vi "WildBugChilGru_V0.195.vi"() -> ()   [LabVIEW 2014]
uses:
  <vilib>/Utility/miscctls.llb/LVPointTypeDef.ctl
  <vilib>/Analysis/NI_AALBase.lvlib
  <vilib>/gmath/NI_Gmath.lvlib
  <vilib>/Analysis/NI_AALPro.lvlib
  <vilib>/Utility/xml.llb/Read From XML File(string).vi
  <vilib>/Utility/xml.llb/Write to XML File(string).vi
  <vilib>/Instr/_visa.llb/VISA Configure Serial Port (Instr).vi
  <vilib>/Analysis/3filter.llb/IIR Filter (DBL).vi
panel:
  in  "Registerkarte":T1(tab)
  in  "Gleitender Mittelwert":u8=35
  in  "Differenzenquotient":u8=12
  in  "Polynom":u8=15
  in  "n vom Gas [1/min]":dbl=5000.0
  in  "Zündung [Imp/U]":u8=5
  in  "Übersetzung ermitteln aus":T2(ring)
  in  "Getriebe [1:]":dbl=5.343
  in  "Reifenumfang [m]":dbl=1.222
  in  "Dauer [s]":dbl=5.0
  in  "nKuWe/nRolle":dbl=10.0
  in  "Rolle [Inkr/U]":u16=10
  in  "Rollenumfang [m]":dbl=0.613
  in  "Rollenträgheit [kgm²]":dbl=0.402
  in  "Lufttemperatur [°C]":dbl=20.0
  in  "Luftfeuchtigkeit [%]":dbl=50.0
  in  "Luftdruck [mbar]":dbl=1013.0
  in  "Messung Klimadaten":bool
  in  "Recalc":bool
  in  "Ende":bool
  out "Datenspeicher":T3
  out "COM-Fehlerrate":string="0 / 0,0%"
  in  "Konfiguration:":bool
  in  "Speichern":bool
  in  "Drucken":bool
  out "Pmax":string="0,0 PS"
  out "Ergebnis":string="0,0 PS bei 0 1/min   |   0,0 Nm bei 0 1/min   |   vmax: 2147483647 km/h\nDIN 70020 k =1,000 (20 °C, 50 %, 1013 mbar)\n20.11.2016 20:05 "
  in  "Fahrzeugdaten":string="Hier die Fahrzeugdaten eingeben"
  out "XY-Graph":cluster{dbl[], dbl[]}[](graph)
  out "Untersetzung\nermittelt":bool
  out "Untersetzung":dbl format="%#.2f"
  in  "Start [F1]":bool
  out "Füllstand Lesepuffer":u64(slide) scale=1.0..100.0
  out "Hinterrad\n[km/h]":dbl(knob) scale=0.0..150.0
  out "Welle\n[1/min]":cluster{dbl, dbl}(knob) scale=0.0..12000.0
  out "Lesepuffer":string="\n"
  in  "Serielle Schnittstelle":refnum<visa-resource-name>="COM6"
  out "Untersetzung-Graph":dbl(graph)=2.6802446808510636 caption="Untersetzung"
  # "1. n konstant halten\n2. START\n3. n weiter halten\n4. bei GO: Vollgas\n5. vom Gas gehen"
  # "Zündung\nRolle"
  # "Untersetzung aus:"
  # "Eingabe <> Messen"
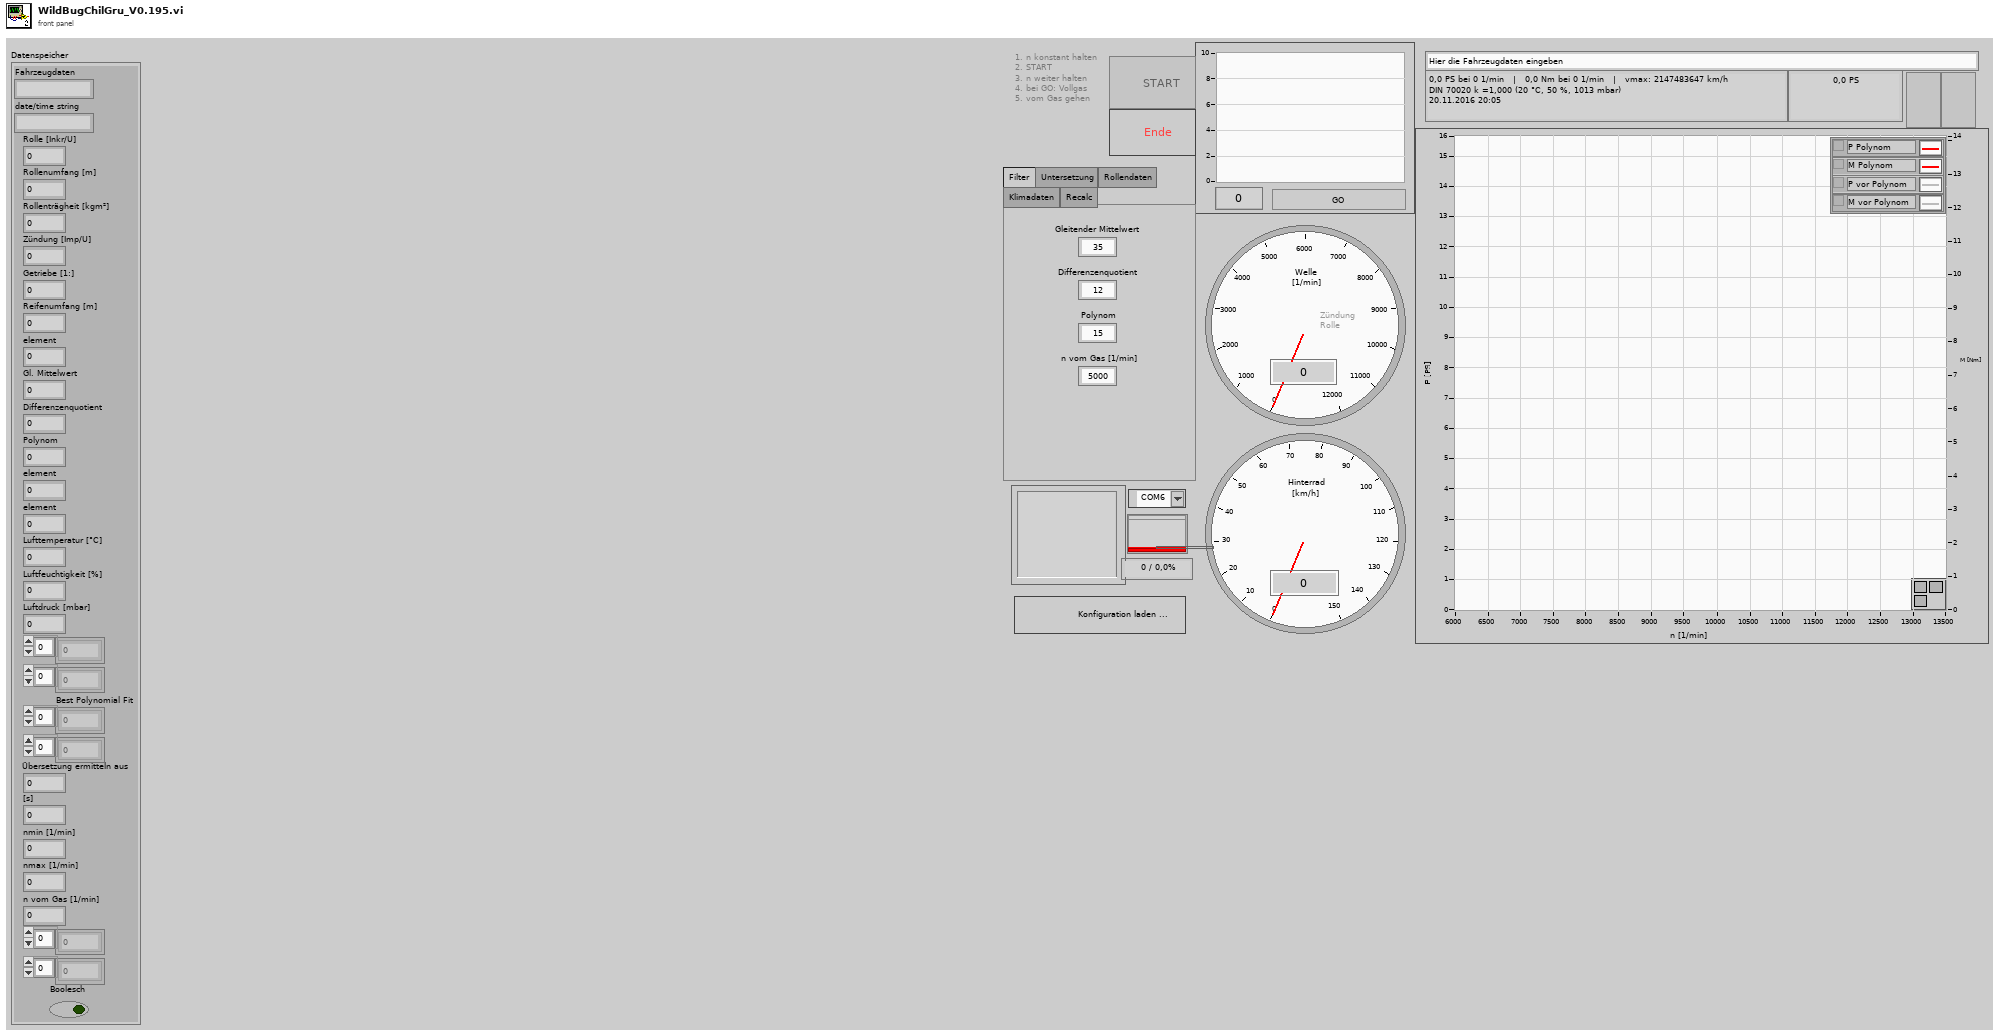
[diagram p1: front panel]
types:
  T1 = enum32{"Filter", "Untersetzung", "Rollendaten", "Klimadaten", "Recalc"}
  T2 = enum8{"Zündsignal", "Getriebe & Reifen", "nKuWe / nRolle"}
  T3 = cluster{"Fahrzeugdaten":string, "date/time string":string, "Rolle [Inkr/U]":u16, "Rollenumfang [m]":dbl, "Rollenträgheit [kgm²]":dbl, "Zündung [Imp/U]":u8, "Getriebe [1:]":dbl, "Reifenumfang [m] ":dbl, "element":dbl, "Gl. Mittelwert":u8, "Differenzenquotient":u8, "Polynom":u8, "element":dbl, "element":dbl, "Lufttemperatur [°C]":dbl, "Luftfeuchtigkeit [%]":dbl, "Luftdruck [mbar]":dbl, dbl[], dbl[], "Best Polynomial Fit":dbl[], dbl[], "Übersetzung ermitteln aus":u8, "[s]":dbl, "nmin [1/min]":dbl, "nmax [1/min]":dbl, "n vom Gas [1/min]":dbl, dbl[], i32[], "Boolesch":bool}
  T4 = enum16{"Kleinste Quadrate", "Kleinestes absolutes Reiduum", "Biquadrat"}
  T5 = enum8{"Enabled", "Disabled", "Disabled and Grayed Out"}
  T6 = cluster{"Fahrzeugdaten":string, "date/time string":string, "Rolle [Inkr/U]":u16, "Rollenumfang [m]":dbl, "Rollenträgheit [kgm²]":dbl, "Zündung [Imp/U]":u8, "Getriebe [1:]":dbl, "Reifenumfang [m] ":dbl, "mean value":dbl, "Gleitender Mittelwert":u8, "Differenzenquotient":u8, "Polynom":u8, dbl, "element":dbl, "Lufttemperatur [°C]":dbl, "Luftfeuchtigkeit [%]":dbl, "Luftdruck [mbar]":dbl, dbl[], dbl[], "Best Polynomial Fit":dbl[], dbl[], "Übersetzung ermitteln aus":enum8{"Zündsignal", "Getriebe & Reifen", "nKuWe / nRolle"}, "Dauer [s]":dbl, dbl, dbl, "n vom Gas [1/min]":dbl, dbl[], i32[], "Messung Klimadaten":bool}
  T7 = typedef "LVPointTypeDef.ctl" = cluster{"Horizontal":i16, "Vertical":i16}
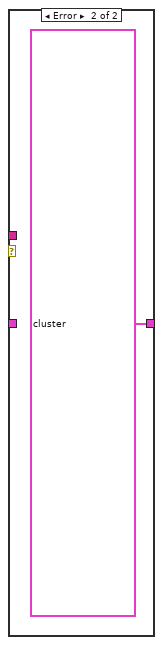
[diagram p2: hidden frame]
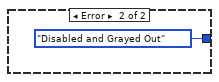
[diagram p3: hidden frame]
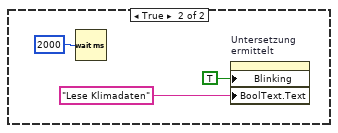
[diagram p5: hidden frame]
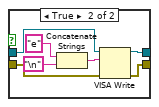
[diagram p6: hidden frame]
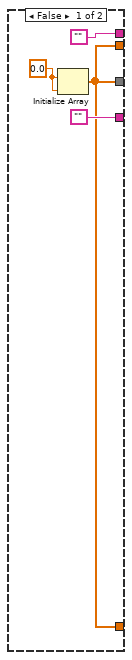
[diagram p8: hidden frame]
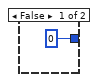
[diagram p9: hidden frame]
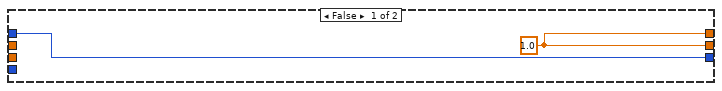
[diagram p11: hidden frame]
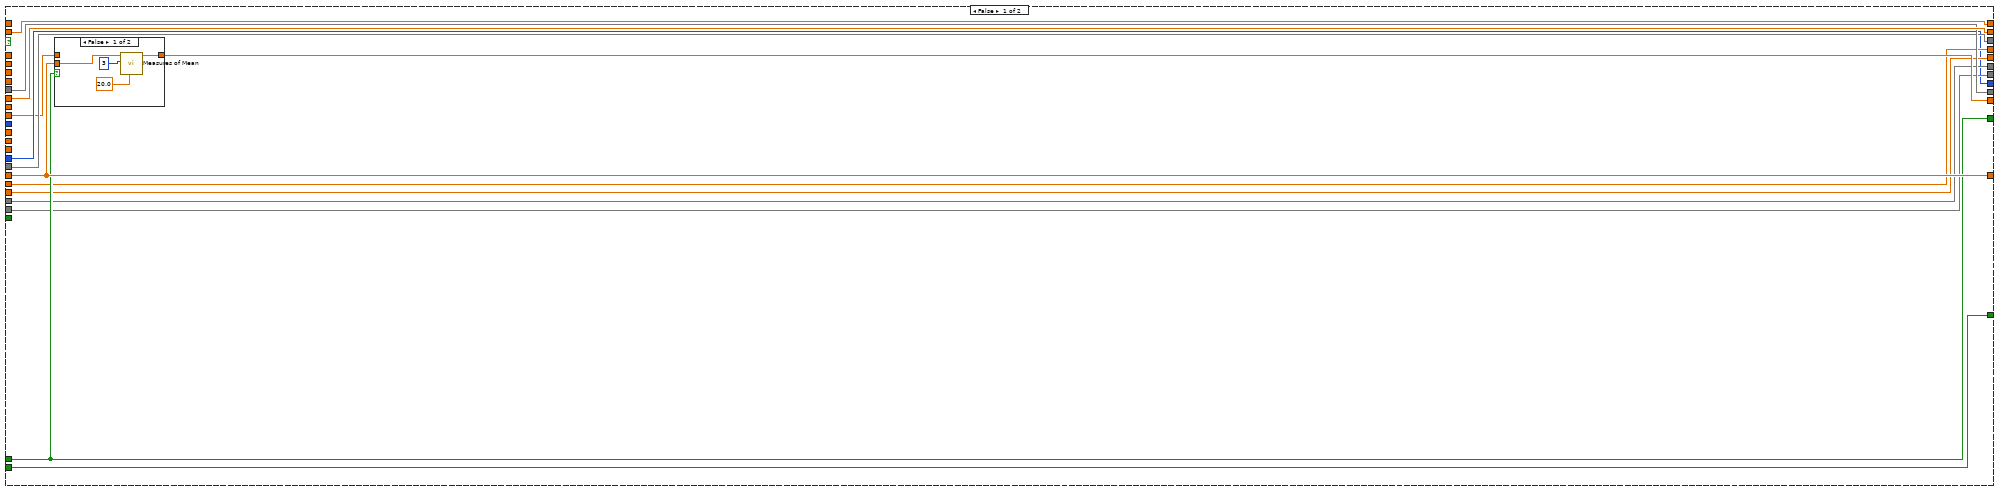
[diagram p12: hidden frame]
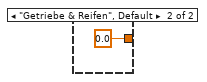
[diagram p16: hidden frame]
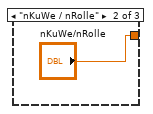
[diagram p18: hidden frame]
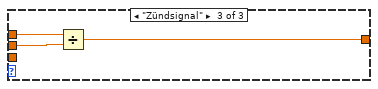
[diagram p19: hidden frame]
diagram:
  n1 = while {
    stop <- w1 stop-if-true
    n2 = event shown="[0] \"Start [F1]\": Wertänderung" {
      selector: _ -> [_ _]
      dyn-events: _ -> [_ _]
      timeout: _ -> [_ _]
      tunnel: [_ TRUE] -> w1
      event "Start [F1]": Value Change {
        n3 = event-data() -> ("NewVal"=w2:bool)  [unwired: 1 in, 5 out]
        n4 = case shown="True" w2 {
          frame False {
          }
          frame True {
            n5 = flat-sequence {
              tunnel: [w132] -> w117
              tunnel: [w131] -> w116
              tunnel: ["Messung Klimadaten"] -> w115
              tunnel: w117 -> [w145]
              tunnel: w116 -> [w144]
              tunnel: [0] -> w114
              tunnel: [1.0 ("element")] -> w113
              tunnel: [w142] -> w112
              tunnel: [w156] -> w111
              tunnel: [0] -> w110
              tunnel: [w142] -> w109
              tunnel: [-5] -> w108
              tunnel: [w153] -> w107
              tunnel: [w151] -> w106
              tunnel: [w150] -> w105
              tunnel: [0.0] -> w104
              tunnel: [w145] -> w103
              tunnel: [w144] -> w102
              tunnel: w115 -> [w143]
              tunnel: [w143] -> w101
              tunnel: w114 -> [w182]
              tunnel: [w182] -> w100
              tunnel: w113 -> [w181]
              tunnel: [w181] -> w99
              tunnel: w112 -> [w180]
              tunnel: [w180] -> w98
              tunnel: w111 -> [w179]
              tunnel: [w179] -> w97
              tunnel: w110 -> [w178]
              tunnel: [w178] -> w96
              tunnel: w109 -> [w177]
              tunnel: [w177] -> w95
              tunnel: w108 -> [w176]
              tunnel: [w176] -> w94
              tunnel: w107 -> [w175]
              tunnel: [w175] -> w93
              tunnel: w106 -> [w174]
              tunnel: [w174] -> w92
              tunnel: w105 -> [w173]
              tunnel: [w173] -> w91
              tunnel: w104 -> [w172]
              tunnel: [w172] -> w90
              tunnel: w103 -> [w171]
              tunnel: [w168] -> w89
              tunnel: w102 -> [w170]
              tunnel: [w169] -> w88
              tunnel: [w167] -> w87
              tunnel: w101 -> [w167]
              tunnel: w100 -> [w206]
              tunnel: [w206] -> w86
              tunnel: w99 -> [w205]
              tunnel: [w205] -> w85
              tunnel: w98 -> [w204]
              tunnel: [w204] -> w84
              tunnel: w97 -> [w203]
              tunnel: [w203] -> w83
              tunnel: w96 -> [w202]
              tunnel: [w202] -> w82
              tunnel: w95 -> [w201]
              tunnel: [w201] -> w81
              tunnel: w94 -> [w200]
              tunnel: [w200] -> w80
              tunnel: w93 -> [w199]
              tunnel: [w199] -> w79
              tunnel: w92 -> [w198]
              tunnel: [w198] -> w78
              tunnel: w91 -> [w197]
              tunnel: [w197] -> w77
              tunnel: w90 -> [w196]
              tunnel: [w196] -> w76
              tunnel: w89 -> [w195]
              tunnel: [w195] -> w75
              tunnel: w88 -> [w194]
              tunnel: [w194] -> w74
              tunnel: w87 -> [w192]
              tunnel: [w192] -> w73
              tunnel: w86 -> [w222]
              tunnel: [w222] -> w72
              tunnel: w85 -> [w221]
              tunnel: [w221] -> w71
              tunnel: w84 -> [w220]
              tunnel: [w220] -> w70
              tunnel: w83 -> [w219]
              tunnel: [w219] -> w69
              tunnel: w82 -> [w218]
              tunnel: [w218] -> w68
              tunnel: w81 -> [w217]
              tunnel: [w217] -> w67
              tunnel: w80 -> [w216]
              tunnel: [w216] -> w66
              tunnel: w79 -> [w215]
              tunnel: [w215] -> w65
              tunnel: w78 -> [w214]
              tunnel: [w214] -> w64
              tunnel: w77 -> [w213]
              tunnel: [w213] -> w63
              tunnel: w76 -> [w212]
              tunnel: [w212] -> w62
              tunnel: w75 -> [w211]
              tunnel: [w210] -> w61
              tunnel: w74 -> [w208]
              tunnel: [w209] -> w60
              tunnel: w73 -> [w207]
              tunnel: w72 -> [w296]
              tunnel: w71 -> [w295]
              tunnel: w70 -> [w294]
              tunnel: w69 -> [w293]
              tunnel: w68 -> [w292]
              tunnel: w67 -> [w291]
              tunnel: w66 -> [w290]
              tunnel: w65 -> [w289]
              tunnel: w64 -> [w288]
              tunnel: w63 -> [w287]
              tunnel: w62 -> [w286]
              tunnel: w61 -> [w251]
              tunnel: [w296] -> w59
              tunnel: [w295] -> w58
              tunnel: [w294] -> w57
              tunnel: [w293] -> w56
              tunnel: [w292] -> w55
              tunnel: [w291] -> w54
              tunnel: [w290] -> w53
              tunnel: [w289] -> w52
              tunnel: [w288] -> w51
              tunnel: [w287] -> w50
              tunnel: [w286] -> w49
              tunnel: [w251] -> w48
              tunnel: [w250] -> w47
              tunnel: [w285] -> w46
              tunnel: [w284] -> w45
              tunnel: [w283] -> w44
              tunnel: ["Gleitender Mittelwert"] -> w43
              tunnel: w60 -> [w250]
              tunnel: [w305] -> w9
              tunnel: [w306] -> w10
              tunnel: [w307] -> w11
              tunnel: [w308] -> w12
              tunnel: [w299] -> w7
              tunnel: [w298] -> w8
              tunnel: [w309] -> w13
              tunnel: [w310] -> w14
              tunnel: [w311] -> w16
              tunnel: [w312] -> w18
              tunnel: [w313] -> w19
              tunnel: [w314] -> w20
              tunnel: [w315] -> w37
              tunnel: [w316] -> w39
              tunnel: [w317] -> w40
              tunnel: [w318] -> w41
              tunnel: [w319] -> w42
              tunnel: w59 -> [w319]
              tunnel: w58 -> [w318]
              tunnel: w57 -> [w317]
              tunnel: w56 -> [w316]
              tunnel: w55 -> [w315]
              tunnel: w54 -> [w314]
              tunnel: w53 -> [w313]
              tunnel: w52 -> [w312]
              tunnel: w51 -> [w311]
              tunnel: w50 -> [w310]
              tunnel: w49 -> [w309]
              tunnel: w48 -> [w301]
              tunnel: w47 -> [w300]
              tunnel: w46 -> [w308]
              tunnel: w45 -> [w307]
              tunnel: w44 -> [w306]
              tunnel: w43 -> [w305]
              frame #0 {
                w137 = u16 0 items=["None", "XON/XOFF", "RTS/CTS", "XON/XOFF & RTS/CTS", "DTR/DSR", "XON/XOFF & DTR/DSR"] ("flow control (0:none)")
                w138 = u16 10 items=["1.0"=10, "1.5"=15, "2.0"=20] ("stop bits (10: 1 bit)")
                w130 = FALSE  # Enable Termination Char (T)
                w133 = u32 10000  # timeout (10sec)
                n6 = call-poly "VISA Configure Serial Port"("VISA resource name"="Serielle Schnittstelle", "timeout (10sec)"=w133, "Enable Termination\nChar (T)"=w130, "baud rate (9600)"=u32 250000 ("baudrate (250000)"), "data bits (8)"=u16 8, "parity (0:none)"=enum16{"None", "Odd", "Even", "Mark", "Space"}."None", "stop bits (10: 1 bit)"=w138, "flow control (0:none)"=w137) -> ("VISA resource name out"=w135:refnum<visa-resource-name>, "error out"=w134:errorcluster)  [unwired: 6 in]
                n7 = VISA Clear(VISA resource name=w135, error in (no error)=w134) -> (VISA resource name out=w132:refnum<visa-resource-name>, error out=w131:errorcluster)
              }
              frame #1 {
                w146 = T5."Disabled and Grayed Out" ("Deaktiviert")
                w149 = 0.0  # Graphen löschen
                w152 = 0
                w157 = 0.0
                w142 = FALSE
                w150 = ""
                n8 = case shown="False" w143 {
                  frame False {
                    n9 = property on="Untersetzung\nermittelt" class="Bool. (strikt)"("Blinking"=TRUE ("Blinkend"), "BoolText.Text"="Initialisiere" ("Beschriftung.Text")) -> ()  [unwired: 2 in, 2 out]
                  }
                  frame True {
                    n10 = Wait (ms)(milliseconds to wait=u32 2000 ("Zu wartende ms")) -> ()  [unwired: 1 out]
                    n11 = property on="Untersetzung\nermittelt" class="Bool. (strikt)"("Blinking"=TRUE ("Blinkend"), "BoolText.Text"="Lese Klimadaten" ("Beschriftung.Text")) -> ()  [unwired: 2 in, 2 out]
                  }
                }
                n12 = Build Array(w149) -> (w148:dbl[])
                n13 = property on="Drucken" class="Bool. (strikt)"("DisabledEnum"=w146) -> ()  [unwired: 2 in, 2 out]
                n14 = property on="Übersetzung ermitteln aus" class="Enum (strikt)"("DisabledEnum"=w146) -> ()  [unwired: 2 in, 2 out]
                n15 = property on="Konfiguration:" class="Bool. (strikt)"("DisabledEnum"=w146) -> ()  [unwired: 2 in, 2 out]
                n16 = property on="Ende" class="Bool. (strikt)"("DisabledEnum"=w146) -> ()  [unwired: 2 in, 2 out]
                n17 = property on="Speichern" class="Bool. (strikt)"("DisabledEnum"=w146) -> ()  [unwired: 2 in, 2 out]
                n18 = property on="Untersetzung-Graph" class="SVDiagr (strikt)"("History Data"=w148) -> ()  [unwired: 2 in, 2 out]
                n19 = local write "Pmax"(w150) -> ()
                n20 = local write "COM-Fehlerrate"(w150) -> ()
                n21 = local write "Ergebnis"(w150) -> ()
                n22 = Initialize Array(w157, w157) -> (w156:dbl[])
                n23 = Initialize Array(w152, w152) -> (w151:i32[])
                n24 = Initialize Array(0.0 ("y"), 0) -> (w153:dbl[])
              }
              frame #2 {
                n25 = case shown="False" w167 {
                  tunnel: w171 -> [w184 w188]
                  tunnel: w170 -> [w183 w187]
                  tunnel: [w183 w186] -> w169
                  tunnel: [w184 w185] -> w168
                  frame False {
                  }
                  frame True {
                    n26 = Concatenate Strings("e" ("String"), "\n") -> (w191:string)
                    n27 = VISA Write(VISA resource name=w188, write buffer=w191, error in (no error)=w187) -> (VISA resource name out=w185:refnum<visa-resource-name>, error out=w186:errorcluster)  [unwired: 1 out]
                  }
                }
              }
              frame #3 {
                n28 = Wait (ms)(milliseconds to wait=u32 500 ("Zu wartende ms")) -> ()  [unwired: 1 out]
              }
              frame #4 {
                n29 = case shown="True" w207 {
                  tunnel: w211 -> [w224 w245]
                  tunnel: [w224 w244] -> w210
                  tunnel: [w223 w243] -> w209
                  tunnel: w208 -> [w223 w242]
                  frame False {
                  }
                  frame True {
                    w227 = ";" ("Regulärer Ausdruck")
                    n30 = property class="Instr"(reference=w245, error in=w242) -> (reference out=w248:refnum<visa-resource-name>, error out=w247:errorcluster, "Serial Settings:Number of Bytes at Serial Port"=w246:u32)
                    n31 = VISA Read(VISA resource name=w248, byte count=w246, error in (no error)=w247) -> (VISA resource name out=w244:refnum<visa-resource-name>, read buffer=w239:string, error out=w243:errorcluster)  [unwired: 1 out]
                    n32 = Search and Replace String(replace all?=TRUE ("Alle ersetzen? (F)"), input string=w239, search string="." ("Such-String"), replace string="," ("Ersetzungs-String (\"\")")) -> (result string=w232:string)  [unwired: 4 in, 3 out]
                    n33 = Match Pattern(string=w232, regular expression=w227) -> (before substring=w230:string, after substring=w231:string)  [unwired: 1 in, 2 out]
                    n34 = Match Pattern(string=w231, regular expression=w227) -> (before substring=w229:string, after substring=w228:string)  [unwired: 1 in, 2 out]
                    n35 = Fract/Exp String To Number(string=w230, offset=1 ("Offset")) -> (number=w238:dbl)  [unwired: 2 in, 1 out]
                    n36 = local write "Lufttemperatur [°C]"(w238) -> ()
                    n37 = Fract/Exp String To Number(string=w229) -> (number=w235:dbl)  [unwired: 3 in, 1 out]
                    n38 = Match Pattern(string=w228, regular expression=w227) -> (before substring=w226:string)  [unwired: 1 in, 3 out]
                    n39 = Fract/Exp String To Number(string=w226) -> (number=w237:dbl)  [unwired: 3 in, 1 out]
                    n40 = Divide(x=w235, y=100.0 ("x")) -> (x/y=w236:dbl)
                    n41 = local write "Luftdruck [mbar]"(w236) -> ()
                    n42 = local write "Luftfeuchtigkeit [%]"(w237) -> ()
                  }
                }
              }
              frame #5 {
                n43 = Wait (ms)(milliseconds to wait=u32 2000 ("Zu wartende ms")) -> ()  [unwired: 1 out]
                n44 = Add(x="Lufttemperatur [°C]", y=273.15) -> (x+y=w266:dbl)
                n45 = Divide ("M_Welle [Nm]")(x=300.0, y=w266) -> (x/y=w269:dbl)
                n46 = Multiply(x="Luftfeuchtigkeit [%]", y=0.01) -> (x*y=w280:dbl)
                n47 = Divide ("M_Welle [Nm]")(x=w266, y=293.15) -> (x/y=w264:dbl)
                n48 = Multiply(x=w280, y=240800000000.0) -> (x*y=w254:dbl)
                n49 = Power Of X(1:w269, 2:5.0) -> (0:w267:dbl)
                n50 = Multiply(x=w254, y=w267) -> (x*y=w274:dbl)
                n51 = Multiply(x=w269, y=-22.644) -> (x*y=w275:dbl)
                n52 = Power Of X(1:w264, 2:0.5) -> (0:w261:dbl)
                n53 = Exponential(1:w275) -> (0:w273:dbl)
                n54 = Multiply(x=w274, y=w273) -> (x*y=w272:dbl)
                n55 = Subtract "p_Trocken [mbar]"(x="Luftdruck [mbar]", y=w272) -> (x-y=w270:dbl)
                n56 = Divide ("M_Welle [Nm]")(x=1013.0, y=w270) -> (x/y=w262:dbl)
                n57 = Multiply "Korrekturfaktor DIN 70020"(x=w262, y=w261) -> (x*y=w285:dbl)
                n58 = Divide(x="Gleitender Mittelwert", y=2) -> (x/y=w258:dbl)
                n59 = Round Toward -Infinity(1:w258) -> (0:w257:dbl)
                n60 = call <vilib>:"Smoothing Filter Coefficients.vi"("shape"=1, "half-width"=w257, "type"=0) -> ("forward coefficients"=w283:dbl[], "reverse coefficients"=w284:dbl[])  [unwired: 6 in, 1 out]
              }
              frame #6 {
                n61 = Concatenate Strings("m" ("String"), "\n") -> (w304:string)
                n62 = property on="Untersetzung\nermittelt" class="Bool. (strikt)"("Blinking"=FALSE ("Blinkend")) -> ()  [unwired: 2 in, 2 out]
                n63 = VISA Write(VISA resource name=w301, write buffer=w304, error in (no error)=w300) -> (VISA resource name out=w298:refnum<visa-resource-name>, error out=w299:errorcluster)  [unwired: 1 out]
              }
            }
            n64 = while {
              tunnel: w8 -> [w450]
              tunnel: w7 -> [w449]
              shift-right: [w520] -> _
              shift-left: w14 -> [w465]
              shift-right: [w515] -> _
              shift-left: w13 -> [w519]
              shift-right: [w514] -> _
              shift-left: w13 -> [w518]
              shift-right: [w469] -> _
              shift-left: w13 -> [w517]
              shift-right: [w496] -> _
              shift-left: w42 -> [w516]
              shift-right: [w457] -> w25
              shift-left: w41 -> [_]
              shift-right: [w475] -> w29
              shift-left: w13 -> [w497]
              shift-right: [w507] -> w27
              shift-left: w13 -> [w471]
              shift-right: [w470] -> _
              shift-left: w18 -> [w511]
              shift-right: [w508] -> _
              shift-left: w40 -> [w485]
              shift-right: [w451] -> _
              shift-left: w39 -> [_]
              shift-right: [w456] -> _
              shift-left: w39 -> [_]
              shift-right: [w506] -> w28
              shift-left: w39 -> [w504]
              shift-right: [w505] -> _
              shift-left: w39 -> [w503]
              shift-right: [w491] -> w36
              shift-left: w18 -> [w502]
              shift-right: [w495] -> _
              shift-left: w18 -> [w500]
              shift-right: [w494] -> w32
              shift-left: w18 -> [w501]
              shift-right: [w493] -> w35
              shift-left: w18 -> [w499]
              shift-right: [w492] -> w34
              shift-left: w18 -> [w498]
              tunnel: [w490] -> w38
              shift-right: [w486] -> w33
              shift-left: w37 -> [w488]
              tunnel: [w489] -> w3
              tunnel: ["n vom Gas [1/min]"] -> w31
              tunnel: ["Rollenumfang [m]"] -> w30
              tunnel: ["Rollenumfang [m]"] -> w24
              shift-right: [w482] -> _
              shift-left: w20 -> [w448]
              shift-right: [w476] -> _
              shift-left: w19 -> [w481]
              shift-right: [w477] -> _
              shift-left: w13 -> [w480]
              shift-right: [w478] -> _
              shift-left: w13 -> [w479]
              shift-right: [w474] -> w17
              shift-left: w18 -> [w473]
              shift-right: [w468] -> _
              shift-left: _ -> [w467]
              shift-right: [w472] -> w15
              shift-left: w16 -> [w466]
              tunnel: [w464] -> w4
              tunnel: w12 -> [w457]
              tunnel: w11 -> [w451]
              tunnel: w10 -> [w456]
              tunnel: w9 -> [w455]
              stop <- w490 stop-if-true
              n65 = property class="Instr"(reference=w450, error in=w449) -> (reference out=w460:refnum<visa-resource-name>, error out=w459:errorcluster, "Serial Settings:Number of Bytes at Serial Port"=w462:u32)
              n66 = Greater?(x=w462, y=u32 1 ("min. Bytes")) -> (0:w458:bool)
              n67 = case shown="True" w458 {
                tunnel: w462 -> [_ w522]
                tunnel: [u32 0 ("Bytes at Port") w522] -> w461
                frame False {
                }
                frame True {
                }
              }
              n68 = case shown="1.." w461 {
                selector: w461 -> [_ w775]
                tunnel: [w725 w769] -> w489
                tunnel: [w724 w770] -> w464
                tunnel: [w729 w771] -> w514
                tunnel: [w730 w768] -> w515
                tunnel: w465 -> [w731 w766]
                tunnel: [w731 w764] -> w520
                tunnel: w519 -> [w730 w756]
                tunnel: w518 -> [w729 w755]
                tunnel: [w726 w754] -> w469
                tunnel: w517 -> [w726 w753]
                tunnel: w516 -> [w728 _]
                tunnel: [w728 w736] -> w496
                tunnel: [w727 w742] -> w468
                tunnel: w467 -> [w727 w741]
                tunnel: w460 -> [w724 w733]
                tunnel: w459 -> [w725 w732]
                frame 0, Default {
                  # "No data in from serial port - Nothing to do."
                }
                frame 1.. {
                  # "Hz Drum"
                  n69 = VISA Read(VISA resource name=w733, byte count=w775, error in (no error)=w732) -> (VISA resource name out=w770:refnum<visa-resource-name>, read buffer=w767:string, error out=w769:errorcluster)  [unwired: 1 out]
                  n70 = Concatenate Strings(w766, w767) -> (w738:string)
                  "Lesepuffer" <- w738
                  n71 = Spreadsheet String To Array(delimiter (Tab)="\n" ("regular expression"), format string="%s" ("regular expression"), spreadsheet string=w738, array type (2D Dbl)=string[] [] ("Array 2")) -> (array=w747:string[])
                  n72 = Match Pattern(string=w738, regular expression="[\\n]") -> (before substring=w745:string, after substring=w765:string, offset past match=w779:i32)  [unwired: 1 in, 1 out]
                  n73 = Array Size(array=w747) -> (size(s)=w751:i32)
                  n74 = Match Pattern(string=w745, regular expression="[;]") -> (before substring=w743:string, after substring=w744:string, offset past match=w740:i32)  [unwired: 1 in, 1 out]
                  n75 = Subtract "aktuelle Zeilenanzahl"(x=w751, y=1) -> (x-y=w736:i32)
                  n76 = property on="Füllstand Lesepuffer" class="Schieber (strikt)"() -> ("Scale.Maximum"=w735:dbl)  [unwired: 2 in, 2 out]
                  n77 = Match Pattern(string=w744, regular expression="[;]") -> (before substring=w774:string, after substring=w777:string, offset past match=w762:i32)  [unwired: 1 in, 1 out]
                  n78 = Match Pattern(string=w777, regular expression="[;]") -> (before substring=w773:string, after substring=w772:string, offset past match=w760:i32)  [unwired: 1 in, 1 out]
                  n79 = Greater Or Equal To 0?(x=w740) -> (x >= 0?=w739:bool)
                  n80 = Greater?(x=w736, y=w735) -> (0:w737:bool)
                  n81 = Greater Or Equal To 0?(x=w760) -> (x >= 0?=w759:bool)
                  n82 = Greater Or Equal To 0?(x=w762) -> (x >= 0?=w761:bool)
                  n83 = Greater Or Equal To 0?(x=w779) -> (x >= 0?=w763:bool)
                  n84 = Select(t=w736, s=w737, f=w735) -> (s? t:f=w734:dbl)
                  n85 = Build Array(w763, w761, w739, w759) -> (w758:bool[])
                  n86 = property on="Füllstand Lesepuffer" class="Schieber (strikt)"("Scale.Maximum"=w734) -> ()  [unwired: 2 in, 2 out]
                  n87 = And Array Elements(Boolean array=w758) -> (logical AND=w757:bool)
                  n88 = case shown="True" w757 {
                    tunnel: w774 -> [_ w790]
                    tunnel: w773 -> [_ w795]
                    tunnel: w772 -> [_ w794]
                    tunnel: [w783 w793] -> w771
                    tunnel: [w784 w792] -> w768
                    tunnel: w765 -> [_ w791]
                    tunnel: [w785 w791] -> w764
                    tunnel: w738 -> [w785 _]
                    tunnel: w756 -> [w784 _]
                    tunnel: w755 -> [w783 _]
                    tunnel: [w782 w789] -> w754
                    tunnel: w753 -> [w782 _]
                    tunnel: w743 -> [_ w788]
                    tunnel: [w781 w786] -> w742
                    tunnel: w741 -> [w781 _]
                    frame False {
                    }
                    frame True {
                      # "Cyclecounter"
                      # "Hz ComLevel"
                      # "ComLevel\nLevel 10 =   6Hz \nLevel 5 =   12Hz \nLevel 4 =   15Hz\nLevel 3 =   20Hz\nLevel 2 =   33Hz\nLevel 1 =   62Hz"
                      # "Hz Drum"
                      # "Hz Engine"
                      # "t4m"
                      n89 = Fract/Exp String To Number(string=w788) -> (number=w787:dbl)  [unwired: 3 in, 1 out]
                      n90 = Fract/Exp String To Number(string=w794) -> (number=w793:dbl)  [unwired: 3 in, 1 out]
                      n91 = Fract/Exp String To Number(string=w790) -> (number=w789:dbl)  [unwired: 3 in, 1 out]
                      n92 = To Long Integer(number=w787) -> (32bit integer=w786:i32)
                      n93 = Fract/Exp String To Number(string=w795) -> (number=w792:dbl)  [unwired: 3 in, 1 out]
                    }
                  }
                }
              }
              "Füllstand Lesepuffer" <- w496
              n94 = Not Equal?(x=w467, y=w468) -> (x != y?=w452:bool)
              n95 = case shown="True" w452 {
                tunnel: w481 -> [w526 w537]
                tunnel: [w526 w549] -> w476
                tunnel: w480 -> [w525 w548]
                tunnel: [w525 w534] -> w477
                tunnel: w479 -> [w524 w547]
                tunnel: [w524 w535] -> w478
                tunnel: w468 -> [_ w533]
                tunnel: w466 -> [w523 w532]
                tunnel: [w523 w536] -> w472
                frame False {
                }
                frame True {
                  n96 = Build Array (concatenate)(w532, w533) -> (w536:i32[])
                  n97 = Greater Or Equal To 0?(x=w537) -> (x >= 0?=w538:bool)
                  n98 = case shown="True" w538 {
                    tunnel: [w550 w561] -> w534
                    tunnel: [w550 w562] -> w535
                    tunnel: [w551 w553] -> w549
                    tunnel: w548 -> [_ w555]
                    tunnel: w547 -> [_ w563]
                    tunnel: w533 -> [w551 w552]
                    tunnel: w537 -> [_ w553]
                    frame False {
                      w550 = 1.0
                    }
                    frame True {
                      w559 = 65536.0
                      n99 = Add(x=w553, y=w555) -> (x+y=w554:dbl)
                      n100 = Divide(x=w554, y=w559) -> (x/y=w564:dbl)
                      n101 = Increment(x=w563) -> (x+1=w562:dbl)
                      n102 = Round Toward -Infinity(1:w564) -> (0:w560:dbl)
                      n103 = Multiply(x=w560, y=w559) -> (x*y=w558:dbl)
                      n104 = Add(x=w558, y=w552) -> (x+y=w557:dbl)
                      n105 = Increment(x=w557) -> (x+1=w556:dbl)
                      n106 = Subtract(x=w556, y=w553) -> (x-y=w561:dbl)
                    }
                  }
                  n107 = Subtract(x=w534, y=w535) -> (x-y=w529:dbl)
                  n108 = Decrement(x=w529) -> (x-1=w528:dbl)
                  n109 = Max & Min(x=0, y=w528) -> (max(x,y)=w527:dbl)  [unwired: 1 out]
                  n110 = Divide(x=w527, y=w534) -> (x/y=w541:dbl)
                  n111 = Greater Than 0?(x=w527) -> (x > 0?=w531:bool)
                  n112 = Select(t=u32 16711680, s=w531, f=u32 0) -> (s? t:f=w542:u32)
                  n113 = Multiply(x=w541, y=100.0) -> (x*y=w539:dbl)
                  n114 = Format Into String(format string="%d / %.1f%%" ("Format-String"), w527, w539) -> (resulting string=→"COM-Fehlerrate":string)  [unwired: 2 in, 1 out]
                  n115 = property on="COM-Fehlerrate" class="Str"("Text.TextColor"=w542) -> ()  [unwired: 2 in, 2 out]
                }
              }
              n116 = case "Case-Struktur" shown="True" w452 {
                tunnel: w515 -> [w705 w716]
                tunnel: w514 -> [w704 w715]
                tunnel: [w705 w714] -> w513
                tunnel: [w704 w713] -> w512
                tunnel: w469 -> [_ w707]
                tunnel: w497 -> [w703 _]
                tunnel: [w703 w706] -> w475
                tunnel: w471 -> [_ w712]
                tunnel: "Rollenumfang [m]" -> [_ w711]
                frame False {
                }
                frame True {
                  w723 = 60.0 ("y")
                  n117 = Reciprocal "Abtastzeit [s]"(x=w707) -> (1/x=w706:dbl)
                  n118 = Divide "R [1/s]"(x=w715, y="Rolle [Inkr/U]") -> (x/y=w722:dbl)
                  n119 = Multiply "nR [1/min]"(x=w723, y=w722) -> (x*y=w713:dbl)
                  n120 = Divide(x=w716, y="Zündung [Imp/U]") -> (x/y=w719:dbl)
                  n121 = Multiply "nZ gemessen [1/min]"(x=w719, y=w723) -> (x*y=w714:dbl)
                  n122 = Multiply "nZ berechnet [1/min]"(x=w713, y=w712) -> (x*y=w721:dbl)
                  n123 = Multiply "[m/min]"(x=w713, y=w711) -> (x*y=w717:dbl)
                  n124 = Multiply "[km/h]"(x=w717, y=0.06) -> (x*y=→"Hinterrad\n[km/h]":dbl)
                  n125 = Bundle(w714, w721) -> (→"Welle\n[1/min]":cluster{dbl, dbl})  [unwired: 1 in]
                }
              }
              n126 = case shown="True" w452 {
                tunnel: w513 -> [_ w634]
                tunnel: w512 -> [_ w633]
                tunnel: "Rollenumfang [m]" -> [_ w637]
                tunnel: [w576 w603] -> w507
                tunnel: w471 -> [w565 w603]
                tunnel: w485 -> [w577 w641]
                tunnel: w511 -> [w578 w640]
                tunnel: [w577 w594] -> w508
                tunnel: [w578 w639] -> w470
                tunnel: w451 -> [_ w636]
                tunnel: w456 -> [_ w635]
                tunnel: [w575 w589] -> w506
                tunnel: [w574 w587] -> w505
                tunnel: w504 -> [w575 w632]
                tunnel: w503 -> [w574 _]
                tunnel: w455 -> [_ w585]
                tunnel: [w573 w609] -> w491
                tunnel: w502 -> [w573 _]
                tunnel: [w572 w624] -> w495
                tunnel: w500 -> [w572 _]
                tunnel: w497 -> [_ w622]
                tunnel: [w571 w610] -> w494
                tunnel: w501 -> [w571 _]
                tunnel: [w570 w626] -> w493
                tunnel: w499 -> [w570 _]
                tunnel: [w569 w625] -> w492
                tunnel: w498 -> [w569 _]
                tunnel: w457 -> [_ w614]
                tunnel: w488 -> [w568 w608]
                tunnel: "n vom Gas [1/min]" -> [_ w596]
                tunnel: [w568 w607] -> w486
                tunnel: w485 -> [_ w606]
                tunnel: w448 -> [w567 w602]
                tunnel: [w567 w601] -> w482
                tunnel: w475 -> [_ w600]
                tunnel: [w566 w599] -> w474
                tunnel: w473 -> [w566 w598]
                frame False {
                  n127 = case shown="False" w577 {
                    tunnel: w578 -> [w582 _]
                    tunnel: [w581 w583] -> w576
                    tunnel: w565 -> [_ w583]
                    frame False {
                      n128 = call <vilib>:"Measures of Mean.vi"("percent (trim)"=20.0, "type"=3, "x array"=w582) -> ("mean value"=w581:dbl)  [unwired: 7 in, 1 out]
                    }
                    frame True {
                    }
                  }
                }
                frame True {
                  w617 = 0.00135962  # [W] in [PS]
                  w628 = 0.10471975511965978  # 2*Pi/60
                  n129 = Build Array (concatenate) "akt. dT in Array einfügen"(w598, w600) -> (w599:dbl[])
                  n130 = Build Array (concatenate) "akt. Rollendrehzahl\nin Array einfügen"(w632, w633) -> (w589:dbl[])
                  n131 = local read "Übersetzung ermitteln aus"() -> (w584:T2)
                  n132 = Index Array(array=w589, index=1 ("Index")) -> (element=w592:dbl)
                  n133 = Initialize Array(w592, w585) -> (w591:dbl[])
                  n134 = case shown="\"Getriebe & Reifen\"" w584 {
                    tunnel: w634 -> [_ _ w702]
                    tunnel: w633 -> [_ _ w701]
                    tunnel: [w697 "nKuWe/nRolle" w700] -> w638
                    tunnel: w637 -> [w698 _ _]
                    frame "Getriebe & Reifen" {
                      n135 = Divide(x=w698, y="Reifenumfang [m]") -> (x/y=w696:dbl)
                      n136 = Multiply(x=w696, y="Getriebe [1:]") -> (x*y=w697:dbl)
                    }
                    frame "nKuWe / nRolle" {
                    }
                    frame "Zündsignal" {
                      n137 = Divide(x=w702, y=w701) -> (x/y=w700:dbl)
                    }
                  }
                  n138 = Insert Into Array(array=w589, index=0 ("Index"), new element=w591) -> (w588:dbl[])
                  n139 = call-poly <vilib>:"IIR Filter.vi"("Forward Coefficients"=w635, "Reverse Coefficients"=w636, "X"=w588) -> ("Filtered X"=w586:dbl[])  [unwired: 1 in, 1 out]
                  n140 = Array Subset(array=w586, index=w585) -> (w587:dbl[])  [unwired: 1 in]
                  n141 = Multiply(x=2.0, y=w622) -> (x*y=w621:dbl)
                  n142 = case shown="False" w641 {
                    selector: w641 -> [_ w693]
                    tunnel: w638 -> [w682 _]
                    tunnel: w640 -> [w684 w692]
                    tunnel: [w678 w693] -> w631
                    tunnel: [w683 w692] -> w639
                    tunnel: w602 -> [w681 w691]
                    tunnel: [w678 w691] -> w601
                    tunnel: w584 -> [w679 _]
                    frame False {
                      n143 = Build Array (concatenate)(w684, w682) -> (w683:dbl[])
                      n144 = case shown="\"Zündsignal\"" w679 {
                        tunnel: ["Dauer [s]" 0.0 ("Dauer [s]")] -> w680
                        frame "Zündsignal" {
                          n145 = property on="Untersetzung\nermittelt" class="Bool. (strikt)"("Blinking"=TRUE ("Blinkend"), "BoolText.Text"="Ermittle Übersetzung" ("Boolescher Text.Text")) -> ()  [unwired: 2 in, 2 out]
                        }
                        frame "Getriebe & Reifen", Default {
                        }
                      }
                      n146 = call "Verstrichene Zeit"("Time Target (s)"=w680, "Reset"=w681) -> ("Time has Elapsed"=w678:bool)  [unwired: 10 in, 7 out]
                      n147 = case shown="True" w678 {
                        frame False {
                        }
                        frame True {
                          n148 = property on="Untersetzung\nermittelt" class="Bool. (strikt)"("Blinking"=FALSE ("Blinkend"), "BoolText.Text"="Go" ("Boolescher Text.Text")) -> ()  [unwired: 2 in, 2 out]
                        }
                      }
                      "Untersetzung-Graph" <- w682
                    }
                    frame True {
                    }
                  }
                  n149 = Array Size "Array-Größe"(array=w587) -> (size(s)=w629:i32)
                  n150 = Square(x=w603) -> (x^2=w627:dbl)
                  n151 = Multiply(x=w587, y=w603) -> (x*y=w609:dbl[])
                  n152 = Multiply(x=w609, y=w628) -> (x*y=w624:dbl[])
                  n153 = Greater?(x=w629, y=w585) -> (0:w630:bool)
                  n154 = Divide(x="Rollenträgheit [kgm²]", y=w627) -> (x/y=w615:dbl)
                  n155 = Multiply(x=w615, y=w614) -> (x*y=w613:dbl)
                  n156 = And(x=w631, y=w630) -> (x .and. y?=w594:bool)
                  n157 = Array Size "Array-Größe"(array=w624) -> (size(s)=w612:i32)
                  n158 = Decrement(x=w612) -> (x-1=w611:i32)
                  n159 = Select(t=w596, s=w594, f=1000000.0) -> (s? t:f=w597:dbl)
                  n160 = Initialize Array(0.0 ("y"), 0) -> (w618:dbl[])
                  n161 = for {
                    N: w612 -> [_]
                    tunnel: "Differenzenquotient" -> [w653]
                    tunnel: w624 -> [w661]
                    tunnel: w611 -> [w652]
                    tunnel: w621 -> [w662]
                    shift-right: [w658] -> w610
                    shift-left: w618 -> [w659]
                    tunnel: w609 -> [w656] mode=indexing
                    tunnel: w608 -> [w644]
                    tunnel: w597 -> [w655]
                    tunnel: [w645] -> w607
                    tunnel: w606 -> [w642]
                    i -> [w646]
                    stop <- w643 stop-if-true
                    n162 = Subtract(x=w652, y=w653) -> (x-y=w654:i32)
                    n163 = Add(x=w646, y=w653) -> (x+y=w669:i32)
                    n164 = Subtract(x=w646, y=w653) -> (x-y=w675:i32)
                    n165 = Greater Or Equal?(x=w646, y=w653) -> (x >= y?=w649:bool)
                    n166 = Greater?(x=w656, y=w655) -> (0:w657:bool)
                    n167 = Max & Min(x=w652, y=w669) -> (min(x,y)=w670:i32)  [unwired: 1 out]
                    n168 = Max & Min(x=w675, y=0) -> (max(x,y)=w673:i32)  [unwired: 1 out]
                    n169 = Subtract(x=w670, y=w646) -> (x-y=w671:i32)
                    n170 = Subtract(x=w646, y=w673) -> (x-y=w672:i32)
                    n171 = Less Or Equal?(x=w646, y=w654) -> (x <= y?=w650:bool)
                    n172 = Max & Min(x=w672, y=w671) -> (min(x,y)=w663:i32)  [unwired: 1 out]
                    n173 = Add(x=w646, y=w663) -> (x+y=w668:i32)
                    n174 = Subtract(x=w646, y=w663) -> (x-y=w667:i32)
                    n175 = Multiply(x=w663, y=w662) -> (x*y=w660:dbl)
                    n176 = Index Array(array=w661, index=w668) -> (element=w665:dbl)
                    n177 = Index Array(array=w661, index=w667) -> (element=w666:dbl)
                    n178 = Subtract(x=w665, y=w666) -> (x-y=w664:dbl)
                    n179 = Divide(x=w664, y=w660) -> (x/y=w651:dbl)
                    n180 = Less Than 0?(x=w651) -> (x < 0?=w648:bool)
                    n181 = Less Or Equal To 0?(x=w644) -> (x <= 0?=w647:bool)
                    n182 = Build Array (concatenate)(w659, w651) -> (w658:dbl[])
                    n183 = Compound Arithmetic op=AND(w648, w657, w647, w649, w650, w642) -> (w643:bool)
                    n184 = case shown="True" w643 {
                      tunnel: w646 -> [_ w677]
                      tunnel: [w676 w677] -> w645
                      tunnel: w644 -> [w676 _]
                      frame False {
                      }
                      frame True {
                      }
                    }
                  }
                  n185 = Multiply(x=w610, y=w613) -> (x*y=w626:dbl[])
                  n186 = Multiply(x=w624, y=w626) -> (x*y=w616:dbl[])
                  n187 = Multiply(x=w617, y=w616) -> (x*y=w625:dbl[])
                }
              }
              "Untersetzung\nermittelt" <- w508
              n188 = local read "Start [F1]"() -> (w454:bool)
              n189 = Greater Than 0?(x=w486) -> (x > 0?=w487:bool)
              n190 = Not(x=w454) -> (.not. x?=w453:bool)
              n191 = Select(t=w507, s=w508, f=0.0) -> (s? t:f=→"Untersetzung":dbl)
              n192 = Or(x=w487, y=w453) -> (x .or. y?=w490:bool)
            }
            n193 = VISA Clear(VISA resource name=w4, error in (no error)=w3) -> (VISA resource name out=w5:refnum<visa-resource-name>, error out=w6:errorcluster)
            n194 = VISA Close(VISA resource name=w5, error in (no error)=w6) -> ()  [unwired: 1 out]
            n195 = case shown="True" w38 {
              tunnel: w36 -> [_ w424]
              tunnel: w35 -> [_ w429]
              tunnel: w34 -> [_ w428]
              tunnel: w33 -> [_ w400]
              tunnel: w32 -> [_ w425]
              tunnel: w31 -> [_ w423]
              tunnel: w30 -> [_ w417]
              tunnel: w25 -> [_ w403]
              tunnel: ["" w402] -> w26
              tunnel: w27 -> [_ w401]
              tunnel: ["" w399] -> _
              tunnel: [w363 w376] -> w23
              tunnel: [w363 w375] -> w22
              tunnel: [w363 w374] -> w21
              frame False {
                w364 = 0.0
                n196 = Initialize Array(w364, w364) -> (w363:dbl[])
              }
              frame True {
                w388 = 735.498  # PS in W
                w394 = 0.10471975511965978  # w = (2 * Pi / 60) * n
                w398 = 0
                n197 = Array Subset "P"(array=w428, length=w400) -> (w420:dbl[])  [unwired: 1 in]
                n198 = Array Subset "M"(array=w429, length=w400) -> (w421:dbl[])  [unwired: 1 in]
                n199 = Array Subset "alpha"(array=w425, length=w400) -> (w426:dbl[])  [unwired: 1 in]
                n200 = Array Subset "n"(array=w424, length=w400) -> (w422:dbl[])  [unwired: 1 in]
                n201 = property on="Ergebnis" class="Str"("Text.FontSize"=18) -> ()  [unwired: 2 in, 2 out]
                n202 = property on="Pmax" class="Str"("Text.FontSize"=48) -> ()  [unwired: 2 in, 2 out]
                n203 = Array Size(array=w426) -> (size(s)=w427:i32)
                n204 = for {
                  N: w427 -> [w447]
                  tunnel: w425 -> [w444]
                  tunnel: w424 -> [w441]
                  tunnel: w423 -> [w438]
                  tunnel: [w436] -> w396
                  i -> [w442]
                  stop <- w437 stop-if-true
                  n205 = Decrement(x=w447) -> (x-1=w446:i32)
                  n206 = Subtract(x=w446, y=w442) -> (x-y=w436:i32)
                  n207 = Index Array(array=w444, index=w436) -> (element=w445:dbl)
                  n208 = Index Array(array=w441, index=w436) -> (element=w440:dbl)
                  n209 = Less?(x=w440, y=w438) -> (x < y?=w439:bool)
                  n210 = Less Or Equal To 0?(x=w445) -> (x <= 0?=w443:bool)
                  n211 = And(x=w443, y=w439) -> (x .and. y?=w437:bool)
                }
                n212 = Increment(x=w396) -> (x+1=w395:i32)
                n213 = Array Subset "P"(array=w420, index=w395) -> (w397:dbl[])  [unwired: 1 in]
                n214 = Array Subset "M"(array=w421, index=w395) -> (w393:dbl[])  [unwired: 1 in]
                n215 = Array Subset "n"(array=w422, index=w395) -> (w376:dbl[])  [unwired: 1 in]
                n216 = Array Max & Min "nmax [1/min]"(array=w376) -> (max value=w419:dbl)  [unwired: 3 out]
                n217 = local write "Polynom"("Polynom") -> ()
                n218 = Bundle(w376, w397) -> (w380:cluster{dbl[], dbl[]})  [unwired: 1 in]
                n219 = Bundle(w376, w393) -> (w381:cluster{dbl[], dbl[]})  [unwired: 1 in]
                n220 = Multiply(x=w376, y=w394) -> (x*y=w390:dbl[])
                n221 = Array Size(array=w376) -> (size(s)=w373:i32)
                n222 = call <vilib>:"General Polynomial Fit.vi"("Y"=w393, "polynomial order"="Polynom", "X"=w376, "method"=T4."Biquadrat" ("Methode"), "algorithm"=3) -> ("Best Polynomial Fit"=w375:dbl[])  [unwired: 7 in, 3 out]
                n223 = Bundle(w376, "Best Polynomial Fit"=w375) -> (w382:cluster{dbl[], "Best Polynomial Fit":dbl[]})  [unwired: 1 in]
                n224 = Multiply(x=w375, y=w390) -> (x*y=w389:dbl[])
                n225 = Multiply(x=w373, y=0.1) -> (x*y=w367:dbl)
                n226 = Multiply(x=w373, y=0.8) -> (x*y=w384:dbl)
                n227 = Array Subset "MPoly ohne die ersten\nund letzten paar %"(array=w375, index=w367, length=w384) -> (w378:dbl[])
                n228 = Array Subset "n ohne die ersten \nund letzten paar %"(array=w376, index=w367, length=w384) -> ()  [unwired: 1 out]
                n229 = Divide(x=w419, y=w401) -> (x/y=w418:dbl)
                n230 = Divide(x=w389, y=w388) -> (x/y=w374:dbl[])
                n231 = Array Subset "PPoly ohne die ersten\nund letzten paar %"(array=w374, index=w367, length=w384) -> (w379:dbl[])
                n232 = Bundle(w376, w374) -> (w383:cluster{dbl[], dbl[]})  [unwired: 1 in]
                n233 = Compound Arithmetic op=MULTIPLY "vmax"(w418, w417, 0.06) -> (w409:dbl)
                n234 = Array Max & Min "Mmax"(array=w378) -> (max value=w386:dbl, max index (indices)=w369:i32)  [unwired: 2 out]
                n235 = Add(x=w367, y=w369) -> (x+y=w368:dbl)
                n236 = Multiply(x=w386, y=1.8) -> (x*y=w430:dbl)
                n237 = Index Array "n(Mmax)"(array=w376, index=w368) -> (element=w410:dbl)
                n238 = Array Max & Min "Pmax"(array=w379) -> (max value=w387:dbl, max index (indices)=w371:i32)  [unwired: 2 out]
                n239 = Build Array(w383, w382, w380, w381) -> (→"XY-Graph":cluster{dbl[], "Best Polynomial Fit":dbl[]}[])
                n240 = Add(x=w367, y=w371) -> (x+y=w370:dbl)
                n241 = local read "Luftfeuchtigkeit [%]"() -> (w413:dbl)
                n242 = local read "Lufttemperatur [°C]"() -> (w412:dbl)
                n243 = local read "Luftdruck [mbar]"() -> (w414:dbl)
                n244 = Multiply(x=w387, y=1.2) -> (x*y=w431:dbl)
                n245 = property on="XY-Graph" class="XYGraph (strikt)"("ActYScl"=1, "YScale.Maximum"=w430, "YScale.Minimum"=w398) -> ()  [unwired: 2 in, 2 out]
                n246 = property on="XY-Graph" class="XYGraph (strikt)"("ActYScl"=w398, "YScale.Maximum"=w431, "YScale.Minimum"=w398) -> ()  [unwired: 2 in, 2 out]
                n247 = Index Array "n(Pmax)"(array=w376, index=w370) -> (element=w415:dbl)
                n248 = Format Into String(format string="%.1f PS" ("Format-String"), w387) -> (resulting string=→"Pmax":string)  [unwired: 2 in, 1 out]
                n249 = Format Date/Time String(time format string (%c)="%x %H:%M ") -> (date/time string=w402:string)  [unwired: 2 in]
                n250 = Format Into String(format string="%.1f PS bei %d 1/min   |   %.1f Nm bei %d 1/min   |   vmax: %d km/h\\nDIN 70020 k =%.3f (%d \\B0C, %d %%, %d mbar)\\n%s" ("Format-String"), w387, w415, w386, w410, w409, w403, w412, w413, w414, w402) -> (resulting string=w399:string)  [unwired: 2 in, 1 out]
                "Ergebnis" <- w399
              }
            }
            n251 = flat-sequence {
              tunnel: w15 -> [w323]
              tunnel: w17 -> [w324]
              tunnel: w21 -> [w325]
              tunnel: w22 -> [w326]
              tunnel: w23 -> [w327]
              tunnel: w24 -> [w328]
              tunnel: w25 -> [w329]
              tunnel: w26 -> [w330]
              tunnel: w27 -> [w331]
              tunnel: w28 -> [w332]
              tunnel: w29 -> [w333]
              tunnel: [w333] -> w128
              tunnel: [w332] -> w127
              tunnel: [w331] -> w126
              tunnel: [w330] -> w125
              tunnel: [w329] -> w124
              tunnel: [w328] -> w123
              tunnel: [w327] -> w122
              tunnel: [w326] -> w121
              tunnel: [w325] -> w120
              tunnel: [w324] -> w119
              tunnel: [w323] -> w118
              tunnel: w128 -> [w362]
              tunnel: w127 -> [w361]
              tunnel: w126 -> [w360]
              tunnel: w125 -> [w359]
              tunnel: w124 -> [w358]
              tunnel: w123 -> [w357]
              tunnel: w122 -> [w356]
              tunnel: w121 -> [w355]
              tunnel: w120 -> [w354]
              tunnel: w119 -> [w353]
              tunnel: w118 -> [w352]
              frame #0 {
                w321 = FALSE ("Start [F1]")
                w322 = 0  # Aktivieren
                n252 = property on="Speichern" class="Bool. (strikt)"("DisabledEnum"=w322) -> ()  [unwired: 2 in, 2 out]
                n253 = property on="Übersetzung ermitteln aus" class="Enum (strikt)"("DisabledEnum"=w322) -> ()  [unwired: 2 in, 2 out]
                n254 = property on="Konfiguration:" class="Bool. (strikt)"("DisabledEnum"=w322) -> ()  [unwired: 2 in, 2 out]
                n255 = property on="Ende" class="Bool. (strikt)"("DisabledEnum"=w322) -> ()  [unwired: 2 in, 2 out]
                n256 = property on="Drucken" class="Bool. (strikt)"("DisabledEnum"=w322) -> ()  [unwired: 2 in, 2 out]
                n257 = property on="Untersetzung\nermittelt" class="Bool. (strikt)"("BoolText.Text"="GO" ("Boolescher Text.Text"), "Blinking"=w321) -> ()  [unwired: 2 in, 2 out]
                n258 = local write "Untersetzung\nermittelt"(w321) -> ()
                n259 = local write "Start [F1]"(w321) -> ()
              }
              frame #1 {
                w336 = 0.0
                n260 = local read "Übersetzung ermitteln aus"() -> (w339:T2)
                n261 = local read "Rollenträgheit [kgm²]"() -> (w349:dbl)
                n262 = local read "Gleitender Mittelwert"() -> (w345:u8)
                n263 = local read "Messung Klimadaten"() -> (w334:bool)
                n264 = local read "Differenzenquotient"() -> (w344:u8)
                n265 = local read "Lufttemperatur [°C]"() -> (w342:dbl)
                n266 = local read "Luftfeuchtigkeit [%]"() -> (w341:dbl)
                n267 = local read "Reifenumfang [m]"() -> (w346:dbl)
                n268 = local read "n vom Gas [1/min]"() -> (w337:dbl)
                n269 = local read "Zündung [Imp/U]"() -> (w348:u8)
                n270 = local read "Luftdruck [mbar]"() -> (w340:dbl)
                n271 = local read "Rolle [Inkr/U]"() -> (w350:u16)
                n272 = local read "Getriebe [1:]"() -> (w347:dbl)
                n273 = local read "Polynom"() -> (w343:u8)
                n274 = local read "Dauer [s]"() -> (w338:dbl)
                n275 = Bundle("Fahrzeugdaten"="Fahrzeugdaten", "date/time string"=w359, "Rolle [Inkr/U]"=w350, "Rollenumfang [m]"=w357, "Rollenträgheit [kgm²]"=w349, "Zündung [Imp/U]"=w348, "Getriebe [1:]"=w347, "Reifenumfang [m]"=w346, "mean value"=w360, "Gleitender Mittelwert"=w345, "Differenzenquotient"=w344, "Polynom"=w343, w362, "element"=w358, "Lufttemperatur [°C]"=w342, "Luftfeuchtigkeit [%]"=w341, "Luftdruck [mbar]"=w340, w361, w356, "Best Polynomial Fit"=w355, w354, "Übersetzung ermitteln aus"=w339, "Dauer [s]"=w338, w336, w336, "n vom Gas [1/min]"=w337, w353, w352, "Messung Klimadaten"=w334) -> (→"Datenspeicher":T6)  [unwired: 1 in]
              }
            }
          }
        }
      }
      event "Ende": Value Change {
        n276 = event-data() -> ()  [unwired: 1 in, 6 out]
      }
    }
  }
  n277 = flat-sequence {
    frame #0 {
      n278 = call <vilib>:"Application Directory.vi"() -> ("Application Directory"=w819:path)
      n279 = Build Path(base path=w819, name or relative path="Konfig.xml") -> (appended path=w817:path)
      n280 = call-poly <vilib>:"Read From XML File.vi"("XML File Path"=w817) -> ("error out"=w798:errorcluster, "XML Elements"=w821:string)  [unwired: 8 in, 1 out]
      n281 = property on="Datenspeicher" class="Cluster (strikt)"() -> ("Value"=w820:T3)  [unwired: 2 in, 2 out]
      n282 = case shown="Kein Fehler" w798 {
        tunnel: w821 -> [w824 _]
        tunnel: w820 -> [w823 _]
        tunnel: [w822 T3 {"Fahrzeugdaten"="", "date/time string"="05.02.2017 22:14 ", "Rolle [Inkr/U]"=10, "Rollenumfang [m]"=0.613, "Rollenträgheit [kgm²]"=0.402, "Zündung [Imp/U]"=5, "Getriebe [1:]"=5.343, "Reifenumfang [m] "=1.222, "element"=2.0, "Gl. Mittelwert"=35, "Differenzenquotient"=12, "Polynom"=15, "element"=0.01639344262295082, "element"=1.0177230216140456, "Lufttemperatur [°C]"=23.3, "Luftfeuchtigkeit [%]"=43.8, "Luftdruck [mbar]"=1013.45, array[1238 elements], array[1224 elements], "Best Polynomial Fit"=array[1224 elements], array[1224 elements], "Übersetzung ermitteln aus"=0, "[s]"=5.0, "nmin [1/min]"=0.0, "nmax [1/min]"=0.0, "n vom Gas [1/min]"=5000.0, array[1238 elements], array[1238 elements], "Boolesch"=TRUE} ("Datenspeicher")] -> w799
        frame No Error {
          n283 = Unflatten From XML(xml string=w824, type=w823) -> (value=w822:T3)  [unwired: 1 in, 1 out]
        }
        frame Error {
        }
      }
      n284 = Unbundle(w799) -> ("Fahrzeugdaten"=w816:string, "Rolle [Inkr/U]"=w815:u16, "Rollenumfang [m]"=w814:dbl, "Rollenträgheit [kgm²]"=w813:dbl, "Zündung [Imp/U]"=w812:u8, "Getriebe [1:]"=w811:dbl, "Reifenumfang [m]"=w810:dbl, "element"=w797:dbl, "Gl. Mittelwert"=w809:u8, "Differenzenquotient"=w808:u8, "Polynom"=w807:u8, "Lufttemperatur [°C]"=w806:dbl, "Luftfeuchtigkeit [%]"=w805:dbl, "Luftdruck [mbar]"=w804:dbl, "Übersetzung ermitteln aus"=w801:u8, "[s]"=w803:dbl, "n vom Gas [1/min]"=w802:dbl, "Boolesch"=w800:bool)  [unwired: 11 out]
      n285 = property on="Datenspeicher" class="Cluster (strikt)"("Value"=w799) -> ()  [unwired: 2 in, 2 out]
      n286 = property on="Polynom" class="DigWert (strikt)"("Value"=w807) -> ()  [unwired: 2 in, 2 out]
      n287 = property on="Dauer [s]" class="DigWert (strikt)"("Value"=w803) -> ()  [unwired: 2 in, 2 out]
      n288 = property on="Fahrzeugdaten" class="Str"("Value"=w816) -> ()  [unwired: 2 in, 2 out]
      n289 = property on="Rolle [Inkr/U]" class="DigWert (strikt)"("Value"=w815) -> ()  [unwired: 2 in, 2 out]
      n290 = property on="Rollenumfang [m]" class="DigWert (strikt)"("Value"=w814) -> ()  [unwired: 2 in, 2 out]
      n291 = property on="Rollenträgheit [kgm²]" class="DigWert (strikt)"("Value"=w813) -> ()  [unwired: 2 in, 2 out]
      n292 = property on="Zündung [Imp/U]" class="DigWert (strikt)"("Value"=w812) -> ()  [unwired: 2 in, 2 out]
      n293 = property on="Getriebe [1:]" class="DigWert (strikt)"("Value"=w811) -> ()  [unwired: 2 in, 2 out]
      n294 = property on="Reifenumfang [m]" class="DigWert (strikt)"("Value"=w810) -> ()  [unwired: 2 in, 2 out]
      n295 = property on="nKuWe/nRolle" class="DigWert (strikt)"("Value"=w797) -> ()  [unwired: 2 in, 2 out]
      n296 = property on="Gleitender Mittelwert" class="DigWert (strikt)"("Value"=w809) -> ()  [unwired: 2 in, 2 out]
      n297 = property on="Differenzenquotient" class="DigWert (strikt)"("Value"=w808) -> ()  [unwired: 2 in, 2 out]
      n298 = property on="Lufttemperatur [°C]" class="DigWert (strikt)"("Value"=w806) -> ()  [unwired: 2 in, 2 out]
      n299 = property on="Luftfeuchtigkeit [%]" class="DigWert (strikt)"("Value"=w805) -> ()  [unwired: 2 in, 2 out]
      n300 = property on="Luftdruck [mbar]" class="DigWert (strikt)"("Value"=w804) -> ()  [unwired: 2 in, 2 out]
      n301 = property on="Übersetzung ermitteln aus" class="Enum (strikt)"("Val(Sgnl)"=w801) -> ()  [unwired: 2 in, 2 out]
      n302 = property on="n vom Gas [1/min]" class="DigWert (strikt)"("Value"=w802) -> ()  [unwired: 2 in, 2 out]
      n303 = property on="Messung Klimadaten" class="Bool. (strikt)"("Val(Sgnl)"=w800) -> ()  [unwired: 2 in, 2 out]
    }
    frame #1 {
      w832 = 2  # Deaktivieren
      w834 = 0.0  # Graphen löschen
      n304 = local read "Serielle Schnittstelle"() -> (w830:refnum<visa-resource-name>)
      n305 = property on="Frontpanel-Position" class="Bereich"("Origin"=T7 {"Horizontal"=8, "Vertical"=6}) -> ()  [unwired: 2 in, 2 out]
      n306 = property on="Füllstand Lesepuffer" class="Schieber (strikt)"("Scale.Maximum"=100) -> ()  [unwired: 2 in, 2 out]
      n307 = property on="Drucken" class="Bool. (strikt)"("DisabledEnum"=w832) -> ()  [unwired: 2 in, 2 out]
      n308 = property on="Speichern" class="Bool. (strikt)"("DisabledEnum"=w832) -> ()  [unwired: 2 in, 2 out]
      n309 = Build Array(w834) -> (w833:dbl[])
      n310 = VISA Clear(VISA resource name=w830) -> (VISA resource name out=w829:refnum<visa-resource-name>, error out=w828:errorcluster)  [unwired: 1 in]
      n311 = property on="Untersetzung-Graph" class="SVDiagr (strikt)"("History Data"=w833) -> ()  [unwired: 2 in, 2 out]
      n312 = VISA Close(VISA resource name=w829, error in (no error)=w828) -> (error out=w827:errorcluster)
      n313 = case shown="Kein Fehler" w827 {
        tunnel: [T5."Enabled" ("Deaktiviert") T5."Disabled and Grayed Out" ("Deaktiviert")] -> w826
        frame No Error {
        }
        frame Error {
        }
      }
      n314 = property on="Start [F1]" class="Bool. (strikt)"("DisabledEnum"=w826) -> ()  [unwired: 2 in, 2 out]
    }
  }
  n315 = while {
    stop <- w838 stop-if-true
    n316 = event shown="[1] \"Drucken\": Wertänderung" {
      selector: _ -> [_ _ _ _ _ _ _ _]
      dyn-events: _ -> [_ _ _ _ _ _ _ _]
      timeout: _ -> [_ _ _ _ _ _ _ _]
      tunnel: [_ _ _ TRUE _ _ _ _] -> w838
      event "Konfiguration:": Value Change {
        n317 = event-data() -> ("OldVal"=w839:bool)  [unwired: 1 in, 5 out]
        n318 = flat-sequence {
          tunnel: [w843] -> w840
          tunnel: w839 -> [w843]
          tunnel: w840 -> [w866]
          frame #0 {
            n319 = call-poly <vilib>:"Read From XML File.vi"() -> ("error out"=w841:errorcluster, "XML Elements"=w844:string)  [unwired: 9 in, 1 out]
            n320 = property on="Datenspeicher" class="Cluster (strikt)"() -> ("Value"=w842:T3)  [unwired: 2 in, 2 out]
            n321 = case shown="Fehler" w841 {
              selector: w841 -> [_ w865]
              tunnel: w844 -> [w864 _]
              tunnel: w842 -> [w863 _]
              frame No Error {
                n322 = Unflatten From XML(xml string=w864, type=w863) -> (value=w862:T3)  [unwired: 1 in, 1 out]
                n323 = Unbundle(w862) -> ("Fahrzeugdaten"=w861:string, "Rolle [Inkr/U]"=w860:u16, "Rollenumfang [m]"=w859:dbl, "Rollenträgheit [kgm²]"=w858:dbl, "Zündung [Imp/U]"=w857:u8, "Getriebe [1:]"=w856:dbl, "Reifenumfang [m]"=w855:dbl, "Gl. Mittelwert"=w854:u8, "Differenzenquotient"=w853:u8, "Polynom"=w852:u8, "Lufttemperatur [°C]"=w851:dbl, "Luftfeuchtigkeit [%]"=w850:dbl, "Luftdruck [mbar]"=w849:dbl, "Übersetzung ermitteln aus"=w846:u8, "[s]"=w848:dbl, "n vom Gas [1/min]"=w847:dbl, "Boolesch"=w845:bool)  [unwired: 12 out]
                n324 = property on="Polynom" class="DigWert (strikt)"("Value"=w852) -> ()  [unwired: 2 in, 2 out]
                n325 = property on="Dauer [s]" class="DigWert (strikt)"("Value"=w848) -> ()  [unwired: 2 in, 2 out]
                n326 = property on="Fahrzeugdaten" class="Str"("Value"=w861) -> ()  [unwired: 2 in, 2 out]
                n327 = property on="Rolle [Inkr/U]" class="DigWert (strikt)"("Value"=w860) -> ()  [unwired: 2 in, 2 out]
                n328 = property on="Rollenumfang [m]" class="DigWert (strikt)"("Value"=w859) -> ()  [unwired: 2 in, 2 out]
                n329 = property on="Rollenträgheit [kgm²]" class="DigWert (strikt)"("Value"=w858) -> ()  [unwired: 2 in, 2 out]
                n330 = property on="Zündung [Imp/U]" class="DigWert (strikt)"("Value"=w857) -> ()  [unwired: 2 in, 2 out]
                n331 = property on="Getriebe [1:]" class="DigWert (strikt)"("Value"=w856) -> ()  [unwired: 2 in, 2 out]
                n332 = property on="Reifenumfang [m]" class="DigWert (strikt)"("Value"=w855) -> ()  [unwired: 2 in, 2 out]
                n333 = property on="Gleitender Mittelwert" class="DigWert (strikt)"("Value"=w854) -> ()  [unwired: 2 in, 2 out]
                n334 = property on="Differenzenquotient" class="DigWert (strikt)"("Value"=w853) -> ()  [unwired: 2 in, 2 out]
                n335 = property on="Lufttemperatur [°C]" class="DigWert (strikt)"("Value"=w851) -> ()  [unwired: 2 in, 2 out]
                n336 = property on="Luftfeuchtigkeit [%]" class="DigWert (strikt)"("Value"=w850) -> ()  [unwired: 2 in, 2 out]
                n337 = property on="Luftdruck [mbar]" class="DigWert (strikt)"("Value"=w849) -> ()  [unwired: 2 in, 2 out]
                n338 = property on="Übersetzung ermitteln aus" class="Enum (strikt)"("Val(Sgnl)"=w846) -> ()  [unwired: 2 in, 2 out]
                n339 = property on="n vom Gas [1/min]" class="DigWert (strikt)"("Value"=w847) -> ()  [unwired: 2 in, 2 out]
                n340 = property on="Messung Klimadaten" class="Bool. (strikt)"("Val(Sgnl)"=w845) -> ()  [unwired: 2 in, 2 out]
              }
              frame Error {
                n341 = call <vilib>:"Clear Errors.vi"("error in (no error)"=w865) -> ()  [unwired: 5 in, 2 out]
              }
            }
          }
          frame #1 {
            n342 = property on="Konfiguration:" class="Bool. (strikt)"("Value"=w866) -> ()  [unwired: 2 in, 2 out]
          }
        }
      }
      event "Drucken": Value Change {
        n343 = event-data() -> ("OldVal"=w867:bool)  [unwired: 1 in, 5 out]
        n344 = flat-sequence {
          tunnel: [w872] -> w868
          tunnel: w867 -> [w872]
          tunnel: w868 -> [w873]
          frame #0 {
            n345 = control-ref of="Fahrzeugdaten"() -> (w870:refnum<vi>)
            n346 = control-ref of="XY-Graph"() -> (w871:refnum<vi>)
            n347 = control-ref of="Ergebnis"() -> (w869:refnum<vi>)
            n348 = call "printgraph_V0.01.vi"("reference 2"=w869, "Fahrzeugdaten"=w870, "XYGraph (Eingang)"=w871) -> ()  [unwired: 9 in]
          }
          frame #1 {
            n349 = property on="Drucken" class="Bool. (strikt)"("Value"=w873) -> ()  [unwired: 2 in, 2 out]
          }
        }
      }
      event "Speichern": Value Change {
        n350 = event-data() -> ("OldVal"=w874:bool)  [unwired: 1 in, 5 out]
        n351 = local write "Speichern"(w874) -> ()
        n352 = local read "Datenspeicher"() -> (w875:T3)
        n353 = Flatten To XML(anything=w875) -> (xml string=w877:string)
        n354 = call-poly <vilib>:"Write to XML File.vi"("XML Input"=w877) -> ("error out"=w876:errorcluster)  [unwired: 8 in, 2 out]
        n355 = case shown="Kein Fehler" w876 {
          frame No Error {
          }
          frame Error {
          }
        }
      }
      event "Ende": Value Change {
        n356 = event-data() -> ("OldVal"=w884:bool)  [unwired: 1 in, 5 out]
        n357 = local write "Ende"(w884) -> ()
        n358 = local read "Datenspeicher"() -> (w881:T3)
        n359 = call <vilib>:"Application Directory.vi"() -> ("Application Directory"=w880:path)
        n360 = Build Path(base path=w880, name or relative path="Konfig.xml") -> (appended path=w878:path)
        n361 = Flatten To XML(anything=w881) -> (xml string=w883:string)
        n362 = call-poly <vilib>:"Write to XML File.vi"("XML Input"=w883, "XML File Path"=w878) -> ("error out"=w882:errorcluster)  [unwired: 7 in, 2 out]
        n363 = case shown="Kein Fehler" w882 {
          frame No Error {
          }
          frame Error {
          }
        }
      }
      event "Serielle Schnittstelle": Value Change {
        n364 = event-data() -> ()  [unwired: 1 in, 6 out]
        n365 = property on="Start [F1]" class="Bool. (strikt)"("DisabledEnum"=T5."Enabled" ("Deaktiviert")) -> ()  [unwired: 2 in, 2 out]
      }
      event "Messung Klimadaten": Value Change {
        n366 = event-data() -> ("NewVal"=w887:bool)  [unwired: 1 in, 5 out]
        n367 = case shown="True" w887 {
          frame True {
            w888 = T5."Disabled and Grayed Out" ("Deaktiviert")
            n368 = property on="Lufttemperatur [°C]" class="DigWert (strikt)"("DisabledEnum"=w888) -> ()  [unwired: 2 in, 2 out]
            n369 = property on="Luftdruck [mbar]" class="DigWert (strikt)"("DisabledEnum"=w888) -> ()  [unwired: 2 in, 2 out]
            n370 = property on="Luftfeuchtigkeit [%]" class="DigWert (strikt)"("DisabledEnum"=w888) -> ()  [unwired: 2 in, 2 out]
          }
          frame False {
            w889 = T5."Enabled" ("Deaktiviert")
            n371 = property on="Lufttemperatur [°C]" class="DigWert (strikt)"("DisabledEnum"=w889) -> ()  [unwired: 2 in, 2 out]
            n372 = property on="Luftdruck [mbar]" class="DigWert (strikt)"("DisabledEnum"=w889) -> ()  [unwired: 2 in, 2 out]
            n373 = property on="Luftfeuchtigkeit [%]" class="DigWert (strikt)"("DisabledEnum"=w889) -> ()  [unwired: 2 in, 2 out]
          }
        }
      }
      event "Recalc": Value Change {
        n374 = event-data() -> ("OldVal"=w892:bool)  [unwired: 1 in, 5 out]
        n375 = property on="Recalc" class="Bool. (strikt)"("Value"=w892) -> ()  [unwired: 2 in, 2 out]
        n376 = property on="Datenspeicher" class="Cluster (strikt)"() -> ("Value"=w891:T3)  [unwired: 2 in, 2 out]
        n377 = call "ReCalc_V0.14.vi"("Berechnen"=TRUE, "Datenspeicher"=w891) -> ()  [unwired: 3 in]
      }
      event "Übersetzung ermitteln aus": Value Change {
        n378 = event-data() -> ("NewVal"=w894:T2)  [unwired: 1 in, 5 out]
        n379 = case shown="\"nKuWe / nRolle\"" w894 {
          tunnel: [T5."Disabled and Grayed Out" ("Deaktiviert") T5."Disabled and Grayed Out" ("Deaktiviert") T5."Enabled" ("Deaktiviert")] -> w896
          frame "nKuWe / nRolle" {
          }
          frame "Zündsignal", Default {
          }
          frame "Getriebe & Reifen" {
          }
        }
        n380 = case shown="\"Zündsignal\", Standard" w894 {
          tunnel: [T5."Enabled" ("Deaktiviert") T5."Disabled and Grayed Out" ("Deaktiviert") T5."Disabled and Grayed Out" ("Deaktiviert")] -> w895
          frame "nKuWe / nRolle" {
          }
          frame "Zündsignal", Default {
          }
          frame "Getriebe & Reifen" {
          }
        }
        n381 = case shown="\"Zündsignal\", Standard" w894 {
          tunnel: [T5."Disabled and Grayed Out" ("Deaktiviert") T5."Enabled" ("Deaktiviert") T5."Disabled and Grayed Out" ("Deaktiviert")] -> w893
          frame "nKuWe / nRolle" {
          }
          frame "Zündsignal", Default {
          }
          frame "Getriebe & Reifen" {
          }
        }
        n382 = property on="Getriebe [1:]" class="DigWert (strikt)"("DisabledEnum"=w896) -> ()  [unwired: 2 in, 2 out]
        n383 = property on="Reifenumfang [m]" class="DigWert (strikt)"("DisabledEnum"=w896) -> ()  [unwired: 2 in, 2 out]
        n384 = property on="nKuWe/nRolle" class="DigWert (strikt)"("DisabledEnum"=w895) -> ()  [unwired: 2 in, 2 out]
        n385 = property on="Dauer [s]" class="DigWert (strikt)"("DisabledEnum"=w893) -> ()  [unwired: 2 in, 2 out]
        n386 = property on="Zündung [Imp/U]" class="DigWert (strikt)"("DisabledEnum"=w893) -> ()  [unwired: 2 in, 2 out]
      }
    }
  }
